vi "test_harness_Sat_op_fxp_16_5.vi"() -> ()   [LabVIEW 2017, in "Sat_Hyst_TestCase.lvclass"]
uses:
  Sat_Hyst_TestCase.lvclass
  C:/Program Files (x86)/National Instruments/LabVIEW 2017/vi.lib/addons/_JKI Toolkits/VI Tester/TestCase.llb/TestCase.lvclass
  hyst_sat_fxp_16_5_weights.ctl
  <vilib>/rvi/DesktopExecutionNode/Execution/niFpgaDEN_Execute.vi
  <vilib>/rvi/DesktopExecutionNode/DesktopExecutionNode.xnode
  <userlib>/_VITAC/VITAC.lvlib
panel:
  out "S_of_uk_fp":sgl[](array[numeric])
  out "Cluster":T1
  in  "Path":path=path "C:/Users/arnold/Documents/matlab/afm_mpc_journal/unit_tests/labview/hyst_sat_data.csv"
  in  "error in (no error)":errorcluster
  out "error out":errorcluster
  out "TestCase out":refnum<class "Sat_Hyst_TestCase.lvclass">
  in  "TestCase in":refnum<class "Sat_Hyst_TestCase.lvclass">
  out "S_of_uk_fxp":fxp<+/-,32,10>[](array[numeric])
  out "S_uk_expected":dbl[](array[numeric])
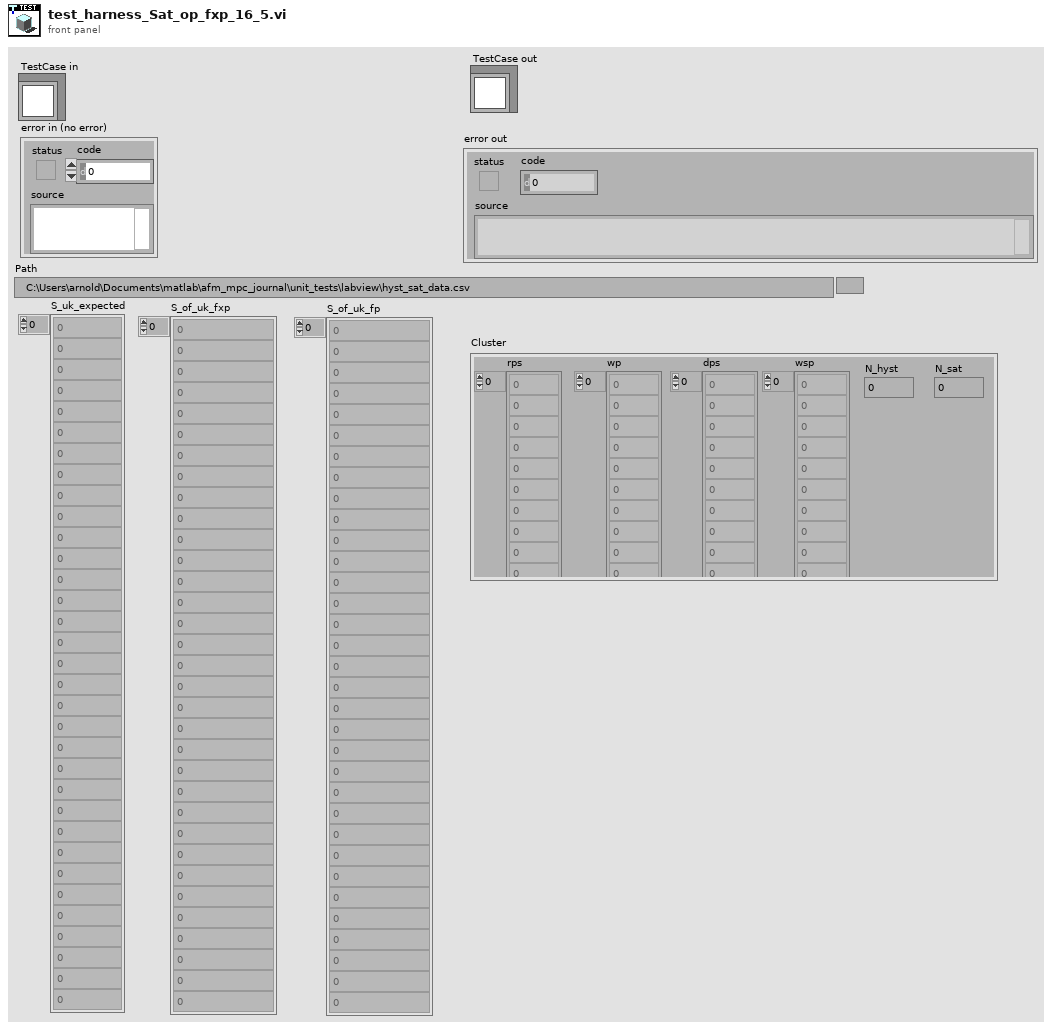
[diagram p1: front panel]
types:
  T1 = typedef "hyst_sat_fxp_16_5_weights.ctl" = cluster{"rps":dbl[], "wp":dbl[], "dps":dbl[], "wsp":dbl[], "N_hyst":i32, "N_sat":i32}
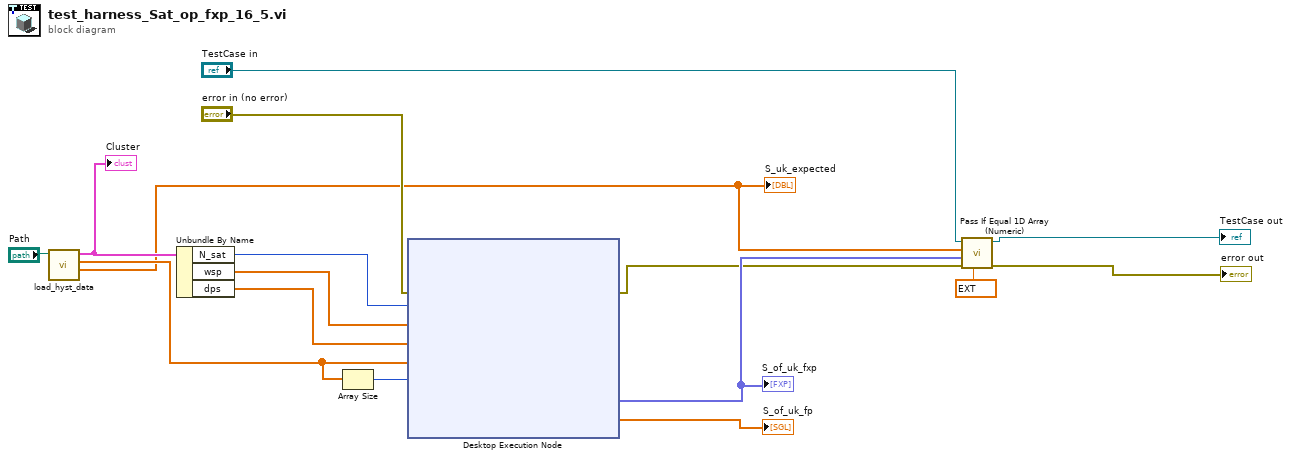
[diagram p0: block diagram]
diagram:
  n1 = call "load_hyst_data.vi"("Path"="Path") -> ("sat_inv(u_nom)"=w2:dbl[], "U_nom"=w3:dbl[], "Cluster"=w7:T1)  [unwired: 6 in, 2 out]
  "S_uk_expected" <- w2
  "Cluster" <- w7
  n2 = Unbundle By Name(w7) -> ("N_sat"=w6:i32, "wsp"=w5:dbl[], "dps"=w4:dbl[])
  n3 = Array Size(array=w3) -> (size(s)=w16:i32)
  n4 = xnode "Desktop Execution Node"("Error In"="error in (no error)", "N_sat"=w6, "satw_s"=w5, "d_s"=w4, "uk"=w3, "numIter"=w16) -> ("Error Out"=w11:errorcluster, "S_of_uk_fxp"=w13:fxp<+/-,32,10>[], "S_of_uk_fp"=→"S_of_uk_fp":sgl[])
  "S_of_uk_fxp" <- w13
  n5 = call <userlib>:"Pass If Equal 1D Array (Numeric).vi"("delta (optional)"=ext 0.00099999999999999999996, "error in (no error)"=w11, "actual"=w13, "expected"=w2, "TestCase in"="TestCase in") -> ("error out"=→"error out":errorcluster, "TestCase out"=→"TestCase out":refnum<class "Sat_Hyst_TestCase.lvclass">)  [unwired: 5 in]
